vi "NicmosSetBankTiming.vi"(0 "error in":errorcluster caption="entrée d'erreur", 2 "Bank Number":i32, 5 "Frame rate":dbl[unit] format="%.2f") -> (3 "error out":errorcluster caption="sortie d'erreur", 6 "Frame rate (out)":dbl[unit] format="%.2f")   [LabVIEW 2009]
doc: "Définition du nombre de lecture du détecteur, de la vitesse de lecture, du mode de lecture et réservation du buffer de lecture associé."
uses:
  NicmosGlobal.vi
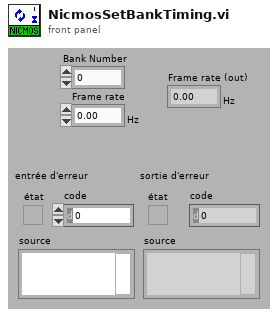
[diagram p1: front panel]
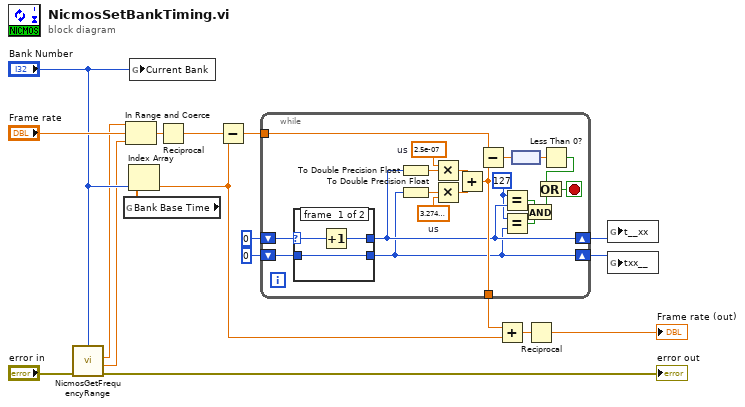
[diagram p0: block diagram]
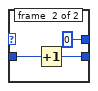
[diagram p2: hidden frame]
diagram:
  n1 = call "NicmosGetFrequencyRange.vi"("Bank Number"="Bank Number", "error in (no error)"="error in") -> ("Max Frame Rate"=w4:dbl[unit], "Min Frame Rate"=w3:dbl[unit], "error out"=→"error out":errorcluster)  [unwired: 5 in]
  n2 = global read "NicmosGlobal.vi" "Bank Base Time"() -> (w7:dbl[unit][])
  n3 = In Range and Coerce(upper limit=w4, x="Frame rate", lower limit=w3) -> (coerced(x)=w6:dbl[unit])  [unwired: 1 out]
  n4 = Index Array(array=w7, index="Bank Number") -> (element=w10:dbl[unit])
  n5 = global write "NicmosGlobal.vi" "Current Bank"("Bank Number") -> ()
  n6 = Reciprocal(x=w6) -> (1/x=w18:dbl[unit])
  n7 = Subtract(x=w18, y=w10) -> (x-y=w15:dbl[unit])
  n8 = while {
    tunnel: [w27] -> w11
    tunnel: w15 -> [w30]
    shift-left: 0 -> [w38]
    shift-right: [w25] -> w8
    shift-left: 0 -> [w37]
    shift-right: [w26] -> w9
    stop <- w20 stop-if-true
    w24 = 127
    w33 = dbl[unit] 3.2749999999999996e-05  # us
    w35 = dbl[unit] 2.5e-07  # us
    n9 = case shown="0, Default" w37 {
      selector: w37 -> [w40 _]
      tunnel: [w39 0] -> w26
      tunnel: w38 -> [w41 w43]
      tunnel: [w41 w42] -> w25
      frame #0 {
        n10 = Increment(x=w40) -> (x+1=w39:i32)
      }
      frame #1 {
        n11 = Increment(x=w43) -> (x+1=w42:i32)
      }
    }
    n12 = To Double Precision Float(number=w26) -> (double precision float=w36:dbl)
    n13 = To Double Precision Float(number=w25) -> (double precision float=w34:dbl)
    n14 = Multiply(x=w35, y=w36) -> (x*y=w32:dbl[unit])
    n15 = Multiply(x=w34, y=w33) -> (x*y=w31:dbl[unit])
    n16 = Add(x=w32, y=w31) -> (x+y=w27:dbl[unit])
    n17 = Subtract(x=w30, y=w27) -> (x-y=w29:dbl[unit])
    n18 = Equal?(x=w24, y=w26) -> (x = y?=w23:bool)
    n19 = Equal?(x=w24, y=w25) -> (x = y?=w22:bool)
    n20 = node(w29) -> (w28:dbl)
    n21 = And(x=w23, y=w22) -> (x .and. y?=w21:bool)
    n22 = Less Than 0?(x=w28) -> (x < 0?=w19:bool)
    n23 = Or(x=w19, y=w21) -> (x .or. y?=w20:bool)
  }
  n24 = Add(x=w11, y=w10) -> (x+y=w12:dbl[unit])
  n25 = Reciprocal(x=w12) -> (1/x=→"Frame rate (out)":dbl[unit])
  n26 = global write "NicmosGlobal.vi" "t__xx"(w9) -> ()
  n27 = global write "NicmosGlobal.vi" "txx__"(w8) -> ()
